vi "Support_Amalgamation.vi"(8 "error in (no error)":errorcluster, 11 "AB_Dest_LLB in":refnum<class "AB_Dest_LLB.lvclass">) -> (0 "error out":errorcluster, 3 "Supports amalgamations?":bool)   [LabVIEW 2020, in "AB_Dest_LLB.lvclass"]
uses:
  <vilib>/AppBuilder/AB_Classes/Destination/Dest_LLB/AB_Dest_LLB.lvclass
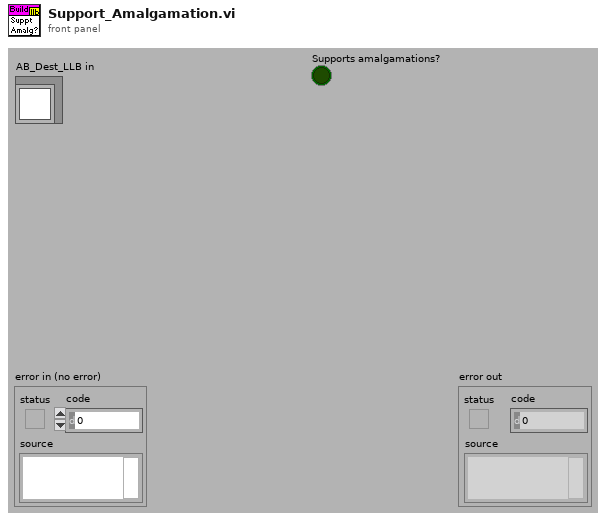
[diagram p1: front panel]
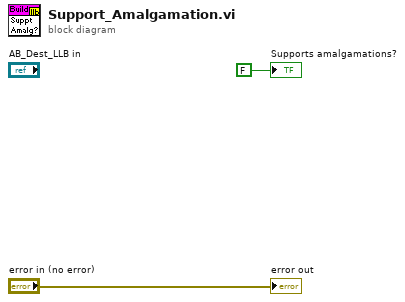
[diagram p0: block diagram]
diagram:
  "error out" <- "error in (no error)"
  "Supports amalgamations?" <- FALSE ("Suppots amalgamations?")
